vi "發牌.vi"() -> ()   [LabVIEW 2015]
panel:
  out "PlayerD":string[](array[string])
  out "PlayerC":string[](array[string])
  out "PlayerB":string[](array[string])
  out "PlayerA":string[](array[string])
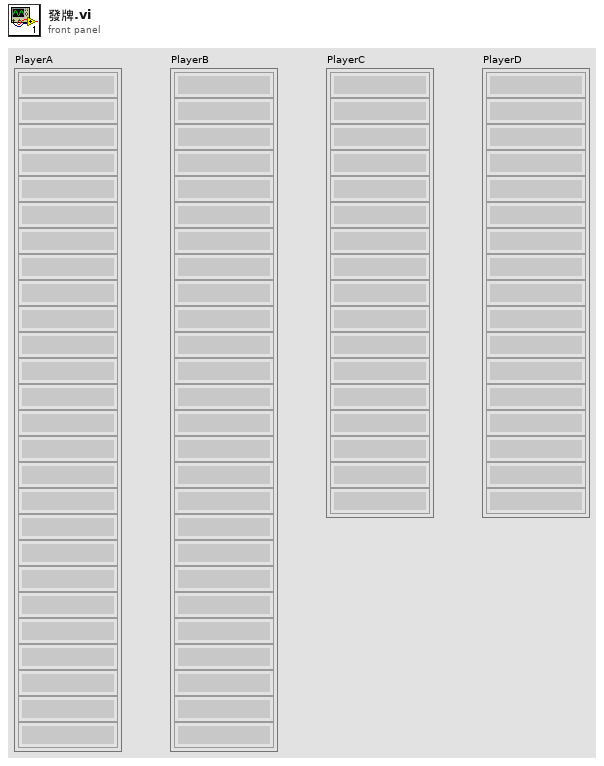
[diagram p1: front panel]
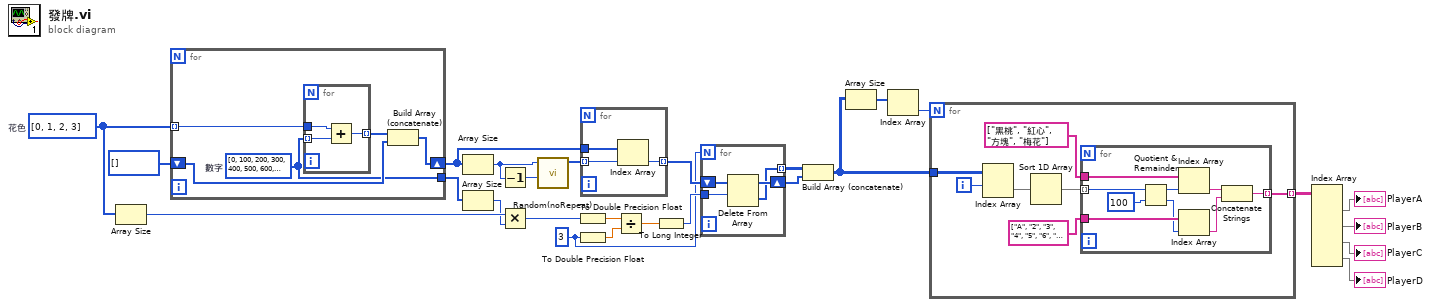
[diagram p0: block diagram]
diagram:
  w4 = 3
  w15 = i32[] [0, 1, 2, 3]  # 花色
  n1 = Array Size(array=w15) -> (size(s)=w13:i32)
  n2 = for {
    tunnel: w15 -> [w31] mode=indexing
    shift-right: [w29] -> w23
    shift-left: i32[] [] -> [w28]
    tunnel: [w27] -> w14
    w27 = i32[] [0, 100, 200, 300, 400, 500, 600, 700, 800, 900, 1000, 1100, 1200]  # 數字
    n3 = for {
      tunnel: w31 -> [w34]
      tunnel: w27 -> [w33] mode=indexing
      tunnel: [w32] -> w30 mode=indexing
      n4 = Add(x=w34, y=w33) -> (x+y=w32:i32)
    }
    n5 = Build Array (concatenate)(w30, w28) -> (w29:i32[])
  }
  n6 = Array Size(array=w23) -> (size(s)=w25:i32)
  n7 = Array Size(array=w14) -> (size(s)=w12:i32)
  n8 = Decrement(x=w25) -> (x-1=w24:i32)
  n9 = Multiply(x=w13, y=w12) -> (x*y=w11:i32)
  n10 = call <userlib>:"Random(noRepeat).vi"("Max"=w24, "輸入點數"=w25) -> ("Array"=w22:i32[])  [unwired: 9 in]
  n11 = To Double Precision Float(number=w11) -> (double precision float=w10:dbl)
  n12 = To Double Precision Float(number=w4) -> (double precision float=w9:dbl)
  n13 = for {
    tunnel: w22 -> [w35] mode=indexing
    tunnel: [w37] -> w21 mode=indexing
    tunnel: w23 -> [w36]
    n14 = Index Array(array=w36, index=w35) -> (element=w37:i32)
  }
  n15 = Divide(x=w10, y=w9) -> (x/y=w7:dbl)
  n16 = To Long Integer(number=w7) -> (32bit integer=w8:i32)
  n17 = for {
    N: w4 -> [_]
    shift-right: [w40] -> w5
    shift-left: w21 -> [w41]
    tunnel: [w39] -> w6 mode=indexing
    tunnel: w8 -> [w38]
    n18 = Delete From Array(array=w41, length=w38) -> (deleted portion=w39:i32[], array with subset deleted=w40:i32[])  [unwired: 1 in]
  }
  n19 = Build Array (concatenate)(w6, w5) -> (w3:i32[][])
  n20 = Array Size(array=w3) -> (size(s)=w2:i32[])
  n21 = Index Array(array=w2) -> (element=w1:i32)  [unwired: 1 in]
  n22 = for {
    N: w1 -> [_]
    tunnel: w3 -> [w48]
    tunnel: [w43] -> w20 mode=indexing
    i -> [w47]
    n23 = Index Array(array=w48, index (row)=w47) -> (element=w46:i32[])  [unwired: 1 in]
    n24 = Sort 1D Array(array=w46) -> (sorted array=w42:i32[])
    n25 = for {
      tunnel: w42 -> [w57] mode=indexing
      tunnel: [w53] -> w43 mode=indexing
      tunnel: string[] ["黑桃", "紅心", "方塊", "梅花"] -> [w52]
      tunnel: string[] ["A", "2", "3", "4", "5", "6", "7", "8", "9", "10", "J", "Q", "K"] -> [w51]
      n26 = Quotient & Remainder(x=w57, y=100) -> (x-y*floor(x/y)=w50:i32, floor(x/y)=w49:i32)
      n27 = Index Array(array=w52, index=w50) -> (element=w55:string)
      n28 = Index Array(array=w51, index=w49) -> (element=w54:string)
      n29 = Concatenate Strings(w55, w54) -> (w53:string)
    }
  }
  n30 = Index Array(array=w20) -> (element #1=→"PlayerA":string[], element #2=→"PlayerB":string[], element #3=→"PlayerC":string[], element #4=→"PlayerD":string[])  [unwired: 8 in]
